vi "1C SmallRCSense.vi"(10 "Wind Direction":T3=45.0 format="%05.1f", 11 "Wind Speed":dbl=1.0) -> (0 "Apparent Wind Speed":T1, 1 "Apparent Wind\nDirection":T2, 2 "Boat\nVelocity":T4 {"East" format="%#_5g"}, 3 "Heading":T3 format="%05.1f", 4 "Eye in the Sky":T6(plugin-control), 5 "Boat Location":T5 {"North" format="%#_10f"; "East" format="%#_8f"})   [LabVIEW 2011]
doc: "Approximates boat location and velocity by tracking visual patterns on a boat seen by a camera. From there, spoofs apparent wind."
uses:
  2-Think/2 Typedefs/UTM Location.ctl
  2-Think/2 Typedefs/Velocity.ctl
  2-Think/2 Typedefs/heading.ctl
  2-Think/2 Typedefs/apparent wind direction.ctl
  2-Think/2 Typedefs/apparent wind speed.ctl
  2-Think/2 Typedefs/pitch and roll.ctl
  2-Think/2 Globals/2 Global.vi
panel:
  out "Frame Rate (Hz)":dbl
  out "Apparent Wind":T4 {"East" format="%#_5g"}
  out "Absolute Wind":T4 {"East" format="%#_5g"}
  in  "Add Randomness\nTo Wind Measurement":bool
  # "TODO: upgrade speed + reliability of pattern matching"
  # "(in boat ref frame)"
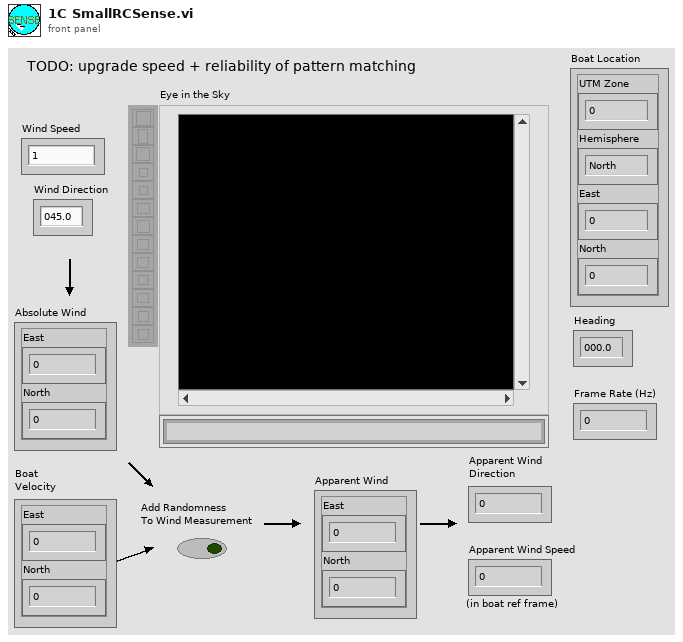
[diagram p1: front panel]
types:
  T1 = typedef "apparent wind speed.ctl" = dbl
  T2 = typedef "apparent wind direction.ctl" = dbl
  T3 = typedef "heading.ctl" = dbl
  T4 = typedef "Velocity.ctl" = cluster{"East":dbl, "North":dbl}
  T5 = typedef "UTM Location.ctl" = cluster{"UTM Zone":dbl, "Hemisphere":enum16{"North", "South"}, "East":dbl, "North":dbl}
  T6 = typedef "IMAQ Image.ctl" = refnum<image>
  T7 = typedef "pitch and roll.ctl" = cluster{"Pitch":dbl, "Roll":dbl}
  T8 = typedef "rate of turn.ctl" = dbl
  T9 = typedef "apparent wind.ctl" = cluster{"Toward Fore":dbl, "Toward Starboard":dbl}
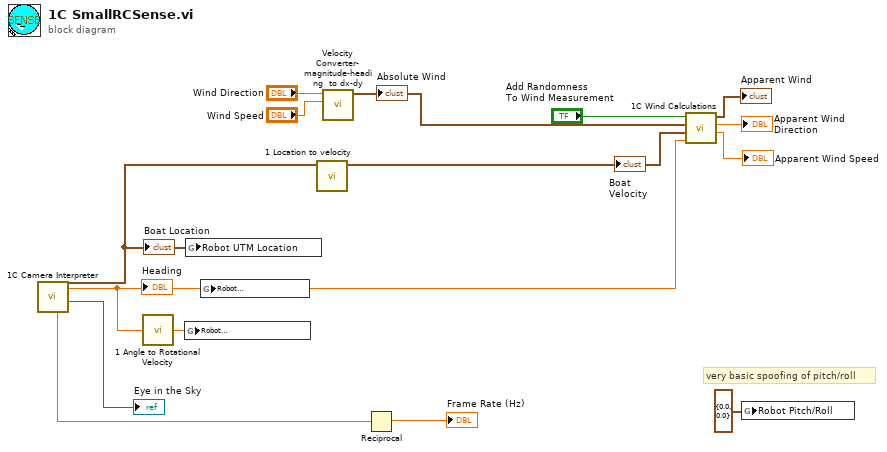
[diagram p0: block diagram]
diagram:
  # "very basic spoofing of pitch/roll"
  n1 = call "1C Camera Interpreter.vi"() -> ("Overhead Image"=→"Eye in the Sky":T6, "Heading"=w1:T3, "Boat Location"=w10:T5, "Time Elapsed (s)\nSince Last Image"=w11:dbl)  [unwired: 7 in, 1 out]
  "Boat Location" <- w10
  "Heading" <- w1
  n2 = call "1 Angle to Rotational Velocity.vi"("Robot\nHeading"=w1) -> ("Robot\nRate of Turn"=w9:T8)
  n3 = global write "2 Global.vi" "Robot\nRate of Turn"(w9) -> ()
  n4 = global write "2 Global.vi" "Robot UTM Location"(w10) -> ()
  n5 = global write "2 Global.vi" "Robot\nHeading"(w1) -> ()
  n6 = call "1 Location to velocity.vi"("Robot UTM Location"=w10) -> ("Velocity"=w7:T4)  [unwired: 10 in]
  "Boat\nVelocity" <- w7
  n7 = call "Velocity Converter- magnitude-heading  to dx-dy.vi"("Magnitude"="Wind Speed", "Heading"="Wind Direction") -> ("Vector Out"=w6:T4)  [unwired: 9 in]
  "Absolute Wind" <- w6
  n8 = Reciprocal(x=w11) -> (1/x=→"Frame Rate (Hz)":dbl)
  n9 = call "1C Wind Calculations.vi"("Boat Heading"=w1, "Boat Velocity"=w7, "Absolute Wind"=w6, "Add Randomness\nTo Wind Measurement"="Add Randomness\nTo Wind Measurement") -> ("Apparent Wind Speed"=→"Apparent Wind Speed":T1, "Apparent Wind\nDirection"=→"Apparent Wind\nDirection":T2, "Apparent Wind"=→"Apparent Wind":T9)  [unwired: 4 in]
  n10 = global write "2 Global.vi" "Robot Pitch/Roll"(T7 {"Pitch"=0.0, "Roll"=0.0} ("Robot Pitch/Roll")) -> ()
